vi "Logrecorder.vi"(1 "error in":errorcluster, 2 "LogPath":path, 3 "Msg":string) -> (0 "error out":errorcluster)   [LabVIEW 2011]
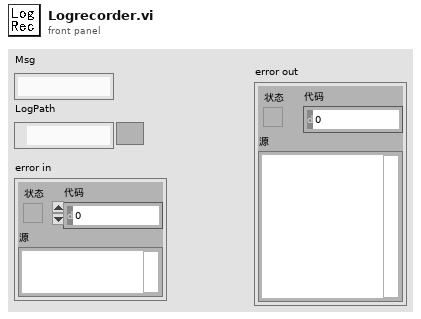
[diagram p1: front panel]
types:
  T1 = enum16{"open", "replace", "create", "open or create", "replace or create", "replace or create with confirmation"}
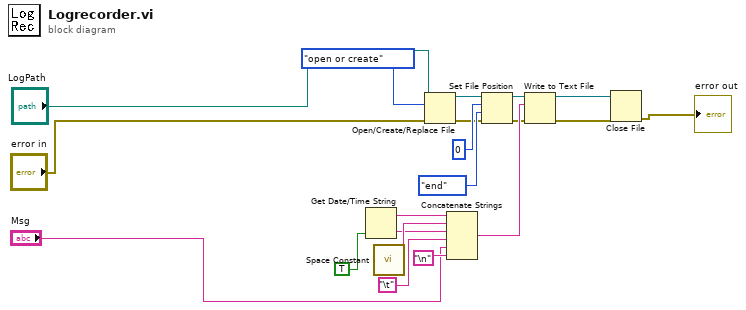
[diagram p0: block diagram]
diagram:
  n1 = Get Date/Time String(want seconds? (F)=TRUE ("需要秒？(F)")) -> (date string=w16:string, time string=w14:string)  [unwired: 2 in]
  n2 = call <vilib>:"Space Constant.vi"() -> ("String"=w15:string)
  n3 = Open/Create/Replace File(file path (use dialog)="LogPath", error in="error in", operation (0:open)=T1."open or create" ("操作(0:open)")) -> (refnum out=w20:refnum<file>, error out=w9:errorcluster)  [unwired: 3 in, 1 out]
  n4 = Concatenate Strings(w16, w15, w14, "\t", "Msg", "\n") -> (w11:string)
  n5 = Set File Position(offset (in bytes) (0)=i64 0 ("偏移量（字节）（0）"), refnum=w20, from (0:start)=enum16{"start", "end", "current"}."end" ("自（0:起始）"), error in=w9) -> (refnum out=w18:refnum<file>, error out=w8:errorcluster)
  n6 = Write to Text File(file (use dialog)=w18, text=w11, error in=w8) -> (refnum out=w6:refnum<file>, error out=w5:errorcluster)  [unwired: 1 in, 1 out]
  n7 = Close File(refnum=w6, error in=w5) -> (error out=→"error out":errorcluster)  [unwired: 1 out]
